vi "Create Status Events.vi"(8 "error in (no error)":errorcluster, 11 "XY Stage Data Class in":refnum<class "XY Stage Data Class.lvclass">) -> (0 "error out":errorcluster, 3 "XY Stage Data Class out":refnum<class "XY Stage Data Class.lvclass">)   [LabVIEW 2022 SP3, in "XY Stage Data Class.lvclass"]
uses:
  XY Stage Data Class.lvclass
  XY Stage Data Class.lvclass/XY Stage Data Class.ctl
  XY Position.ctl
  Moving.ctl
  Homed.ctl
  Current Speed.ctl
  Acceleration.ctl
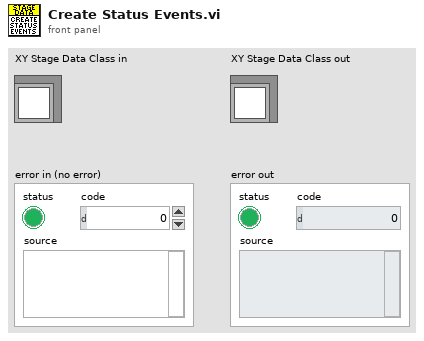
[diagram p1: front panel]
types:
  T1 = typedef "XY Stage Data Class.lvclass/Acceleration.ctl" = cluster{"X Acceleration":dbl, "Y Acceleration":dbl}
  T2 = typedef "XY Stage Data Class.lvclass/Current Speed.ctl" = cluster{"X Current Speed":dbl, "Y Current Speed":dbl}
  T3 = typedef "XY Stage Data Class.lvclass/Homed.ctl" = cluster{"X Homed":bool, "Y Homed":bool}
  T4 = typedef "XY Stage Data Class.lvclass/Moving.ctl" = cluster{"X Moving":bool, "Y Moving":bool}
  T5 = typedef "XY Stage Data Class.lvclass/XY Position.ctl" = cluster{"Current Position X":dbl, "Current Position Y":dbl}
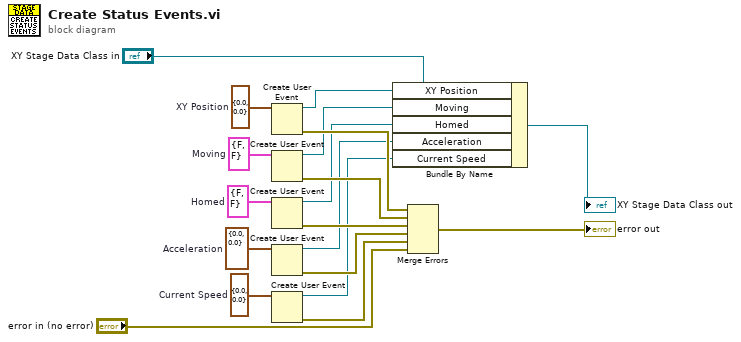
[diagram p0: block diagram]
diagram:
  w3 = T1 {"X Acceleration"=0.0, "Y Acceleration"=0.0}  # Acceleration
  w2 = T2 {"X Current Speed"=0.0, "Y Current Speed"=0.0}  # Current Speed
  w4 = T3 {"X Homed"=FALSE, "Y Homed"=FALSE}  # Homed
  w5 = T4 {"X Moving"=FALSE, "Y Moving"=FALSE}  # Moving
  w6 = T5 {"Current Position X"=0.0, "Current Position Y"=0.0}  # XY Position
  n1 = Create User Event(user event datatype=w6) -> (user event=w12:refnum<user-event>, error out=w13:errorcluster)  [unwired: 1 in]
  n2 = Create User Event(user event datatype=w5) -> (user event=w11:refnum<user-event>, error out=w14:errorcluster)  [unwired: 1 in]
  n3 = Create User Event(user event datatype=w4) -> (user event=w10:refnum<user-event>, error out=w15:errorcluster)  [unwired: 1 in]
  n4 = Create User Event(user event datatype=w3) -> (user event=w9:refnum<user-event>, error out=w16:errorcluster)  [unwired: 1 in]
  n5 = Create User Event(user event datatype=w2) -> (user event=w8:refnum<user-event>, error out=w17:errorcluster)  [unwired: 1 in]
  n6 = Bundle By Name(cluster="XY Stage Data Class in", "XY Position"=w12, "Moving"=w11, "Homed"=w10, "Acceleration"=w9, "Current Speed"=w8) -> (→"XY Stage Data Class out":refnum<class "XY Stage Data Class.lvclass">)
  n7 = Merge Errors(w13, w14, w15, w16, w17, "error in (no error)") -> (→"error out":errorcluster)
